vi "Main Window.vi"() -> ()   [LabVIEW 2015]
uses:
  Control Button/Exit.ctl
  Control Button/login.ctl
  Control Button/Logout.ctl
  Control Button/setting.ctl
  Control Button/report.ctl
  Control Button/Manual.ctl
  Control Button/Start.ctl
  Enqueue/Main window Seq/Test selection_1.ctl
  Enqueue/Main window Seq/Test seq_1.ctl
  Galobal variable_TI.vi
  Project Setup/Globle Variable/GR_Servo.vi
panel:
  out "User Name":string
  out "error out":errorcluster
  out "x = y?":bool
  out "Company Name":string
  in  "Sign In":T1
  out "Boolean":bool
  in  "Dashbord":T6
  in  "Login Window":T8 {"User Name" items=["admin", "mmum", "a", "AJAY Kumar", "", "", "", "", "", "", "", "", "", "", "", "", "", "", "", "", "", "", "", "", "", "", "", "", "", "", "", ""]}
  in  "Exit":T9
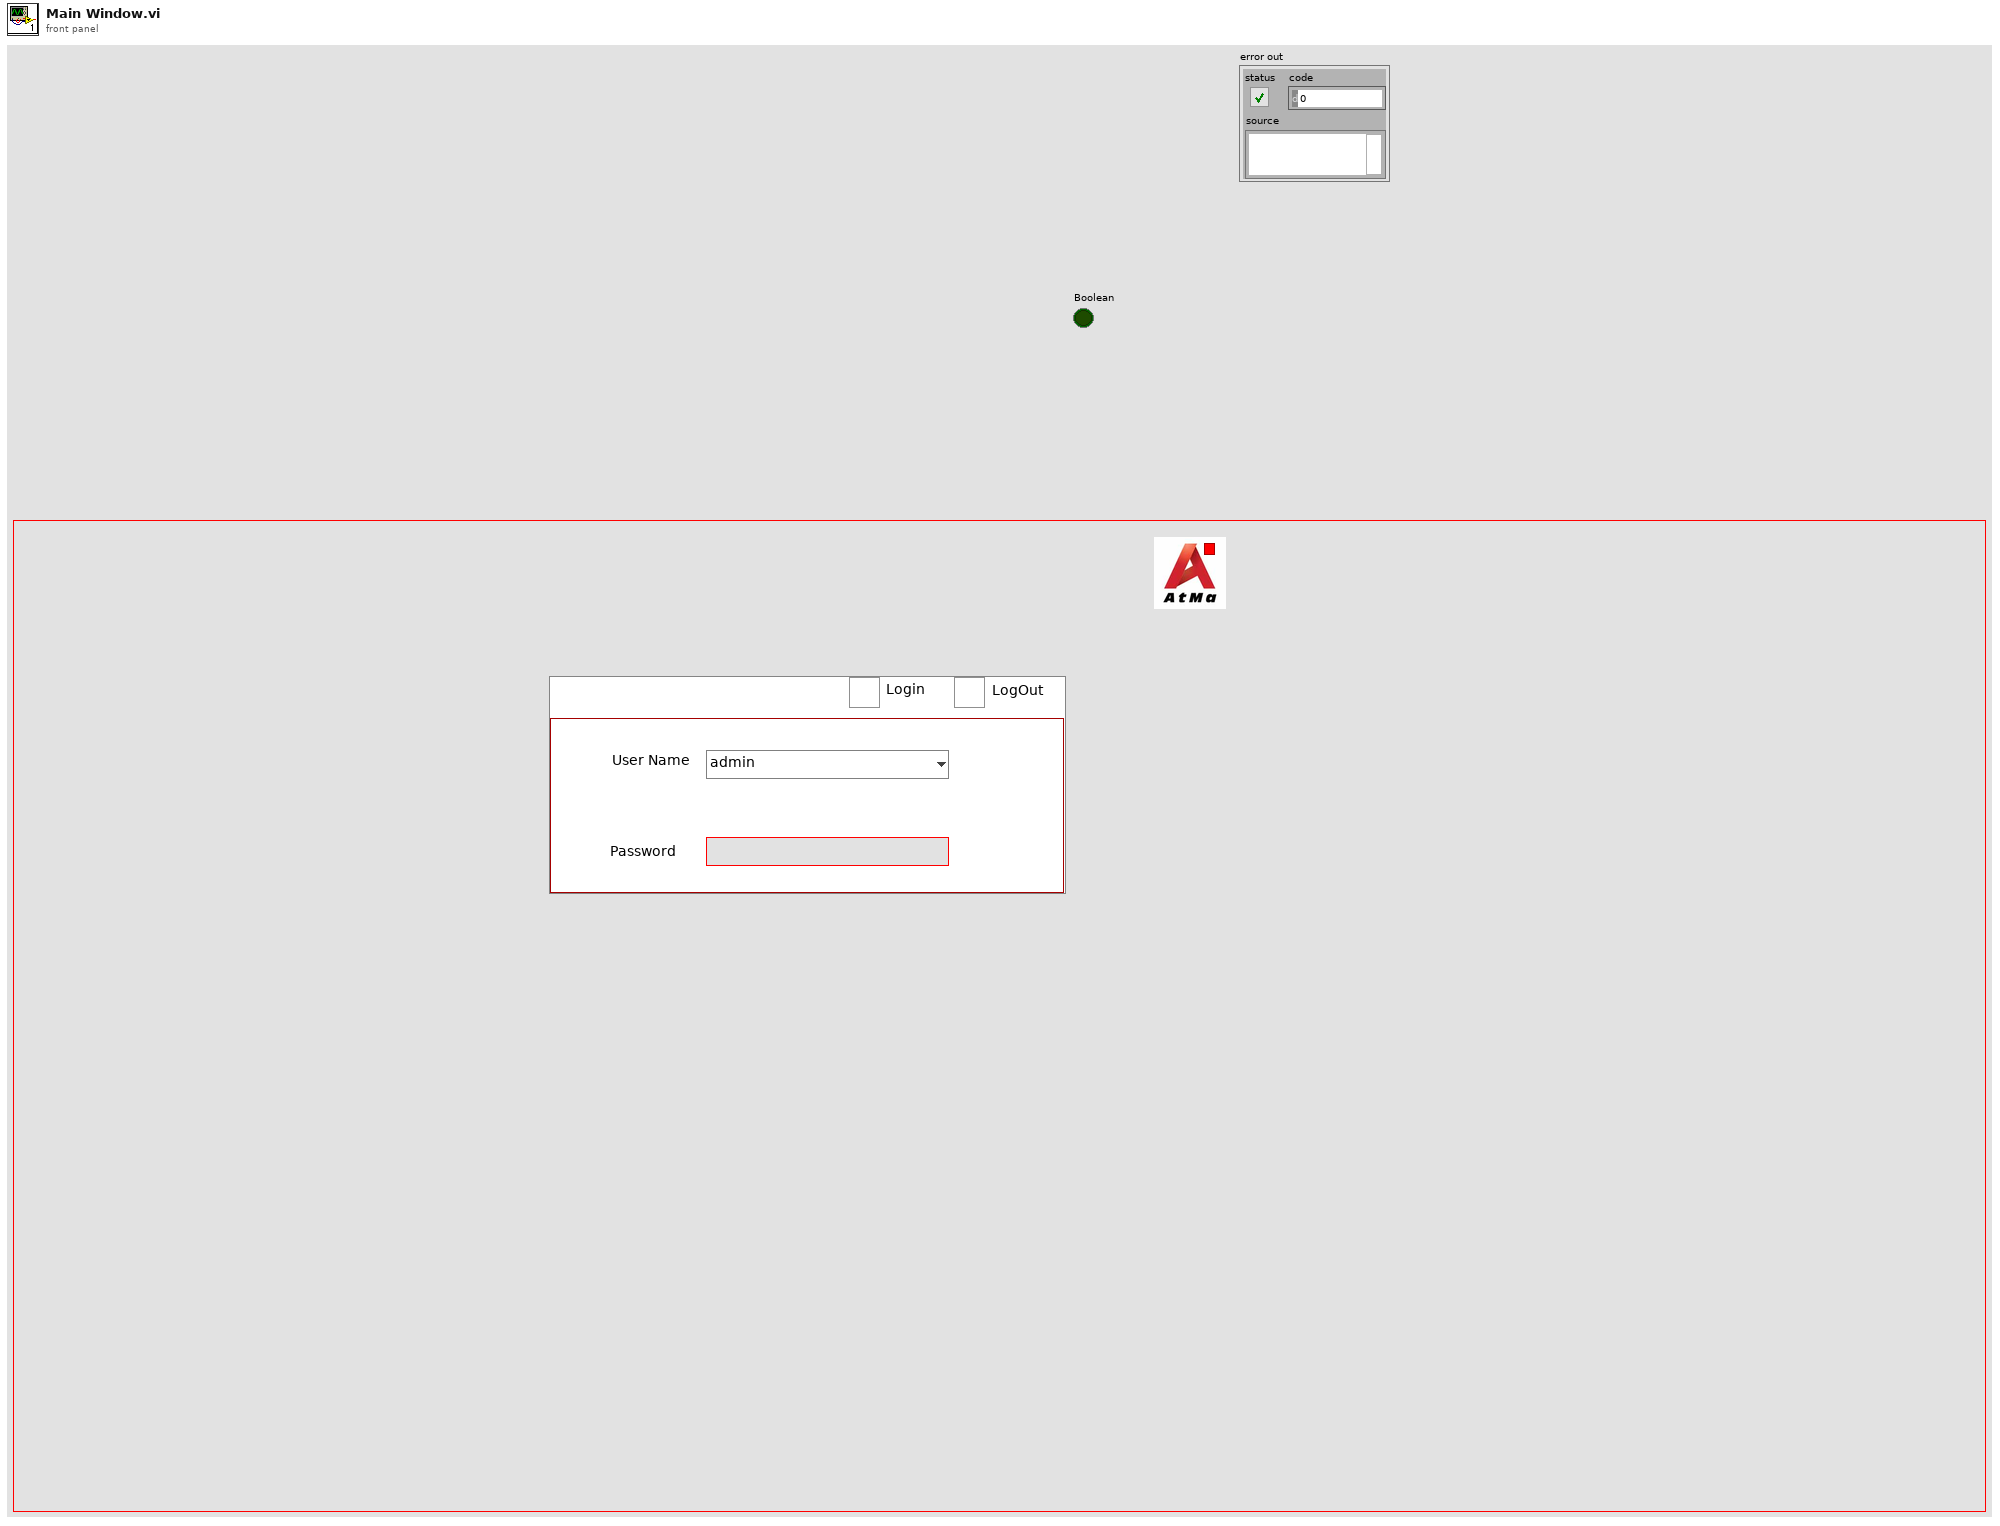
[diagram p1: front panel]
types:
  T1 = typedef "login.ctl" = bool
  T2 = typedef "setting.ctl" = bool
  T3 = typedef "report.ctl" = bool
  T4 = typedef "Manual.ctl" = bool
  T5 = typedef "Start.ctl" = bool
  T6 = cluster{"Setting":T2, "Report":T3, "Manaul":T4, "Start":T5}
  T7 = typedef "Logout.ctl" = bool
  T8 = cluster{"User Name":u16, "Password":string, "Sign In":T1, "Log Out":T7}
  T9 = typedef "Exit.ctl" = bool
  T10 = typedef "Test selection_1.ctl" = enum16{"Init", "Enqueue ", "Enqueue N", "Enqueue in stack", "Enqueue in stack N", "Dequeue", "Dequeue N", "Flush", "Release Queue"}
  T11 = typedef "Test seq_1.ctl" = enum16{"Poll Event", "Login", "Logout", "Confi", "Manual", "Report", "Testing", "Exit"}
  T12 = cluster{"XInput":dbl[], "Y New Value":dbl[], "Avg point":i16}[]
  T13 = cluster{"Slop":dbl[], "Intercept":dbl[], "Average ":i16[]}
  T14 = cluster{"UserName":string[], "Password":string[], "Usertype":string[], "Analog Min":string[], "Analog Max":string[], "DigitalInput Port":string[], "Digital Output Port":string[], "ANalog Port":string[], "IOList":cluster{"DI List_280":string[], "D0List _280":string[], "AI List_280":string[]}}
  T15 = cluster{"DI List_280":string[], "D0List _280":string[], "AI List_280":string[]}
  T16 = cluster{"DigitalInput Port[0]":string, "DigitalInput Port[1]":string, "DigitalInput Port[2]":string, "DigitalInput Port[3]":string, "DigitalInput Port[4]":string, "DigitalInput Port[5]":string, "DigitalInput Port[6]":string, "DigitalInput Port[7]":string, "DigitalInput Port[8]":string, "DigitalInput Port[9]":string, "DigitalInput Port[10]":string, "DigitalInput Port[11]":string, "DigitalInput Port[12]":string, "DigitalInput Port[13]":string, "DigitalInput Port[14]":string, "DigitalInput Port[15]":string}
  T17 = cluster{"Digital Output Port[0]":string, "Digital Output Port[1]":string, "Digital Output Port[2]":string, "Digital Output Port[3]":string, "Digital Output Port[4]":string, "Digital Output Port[5]":string, "Digital Output Port[6]":string, "Digital Output Port[7]":string, "Digital Output Port[8]":string, "Digital Output Port[9]":string, "Digital Output Port[10]":string, "Digital Output Port[11]":string, "Digital Output Port[12]":string, "Digital Output Port[13]":string, "Digital Output Port[14]":string, "Digital Output Port[15]":string, "Digital Output Port[16]":string, "Digital Output Port[17]":string, "Digital Output Port[18]":string, "Digital Output Port[19]":string, "Digital Output Port[20]":string, "Digital Output Port[21]":string, "Digital Output Port[22]":string, "Digital Output Port[23]":string, "Digital Output Port[24]":string, "Digital Output Port[25]":string, "Digital Output Port[26]":string, "Digital Output Port[27]":string, "Digital Output Port[28]":string, "Digital Output Port[29]":string}
  T18 = cluster{"ANalog Port[0]":string, "ANalog Port[1]":string, "ANalog Port[2]":string, "ANalog Port[3]":string, "ANalog Port[4]":string, "ANalog Port[5]":string, "ANalog Port[6]":string, "ANalog Port[7]":string, "ANalog Port[8]":string, "ANalog Port[9]":string, "ANalog Port[10]":string, "ANalog Port[11]":string, "ANalog Port[12]":string, "ANalog Port[13]":string, "ANalog Port[14]":string, "ANalog Port[15]":string, "ANalog Port[16]":string, "ANalog Port[17]":string, "ANalog Port[18]":string, "ANalog Port[19]":string, "ANalog Port[20]":string, "ANalog Port[21]":string, "ANalog Port[22]":string, "ANalog Port[23]":string, "ANalog Port[24]":string, "ANalog Port[25]":string, "ANalog Port[26]":string, "ANalog Port[27]":string, "ANalog Port[28]":string, "ANalog Port[29]":string, "ANalog Port[30]":string, "ANalog Port[31]":string}
  T19 = enum32{"Invalid", "Standard", "Closed", "Hidden", "Minimized", "Maximized"}
  T20 = enum8{"Enabled", "Disabled", "Disabled and Grayed Out"}
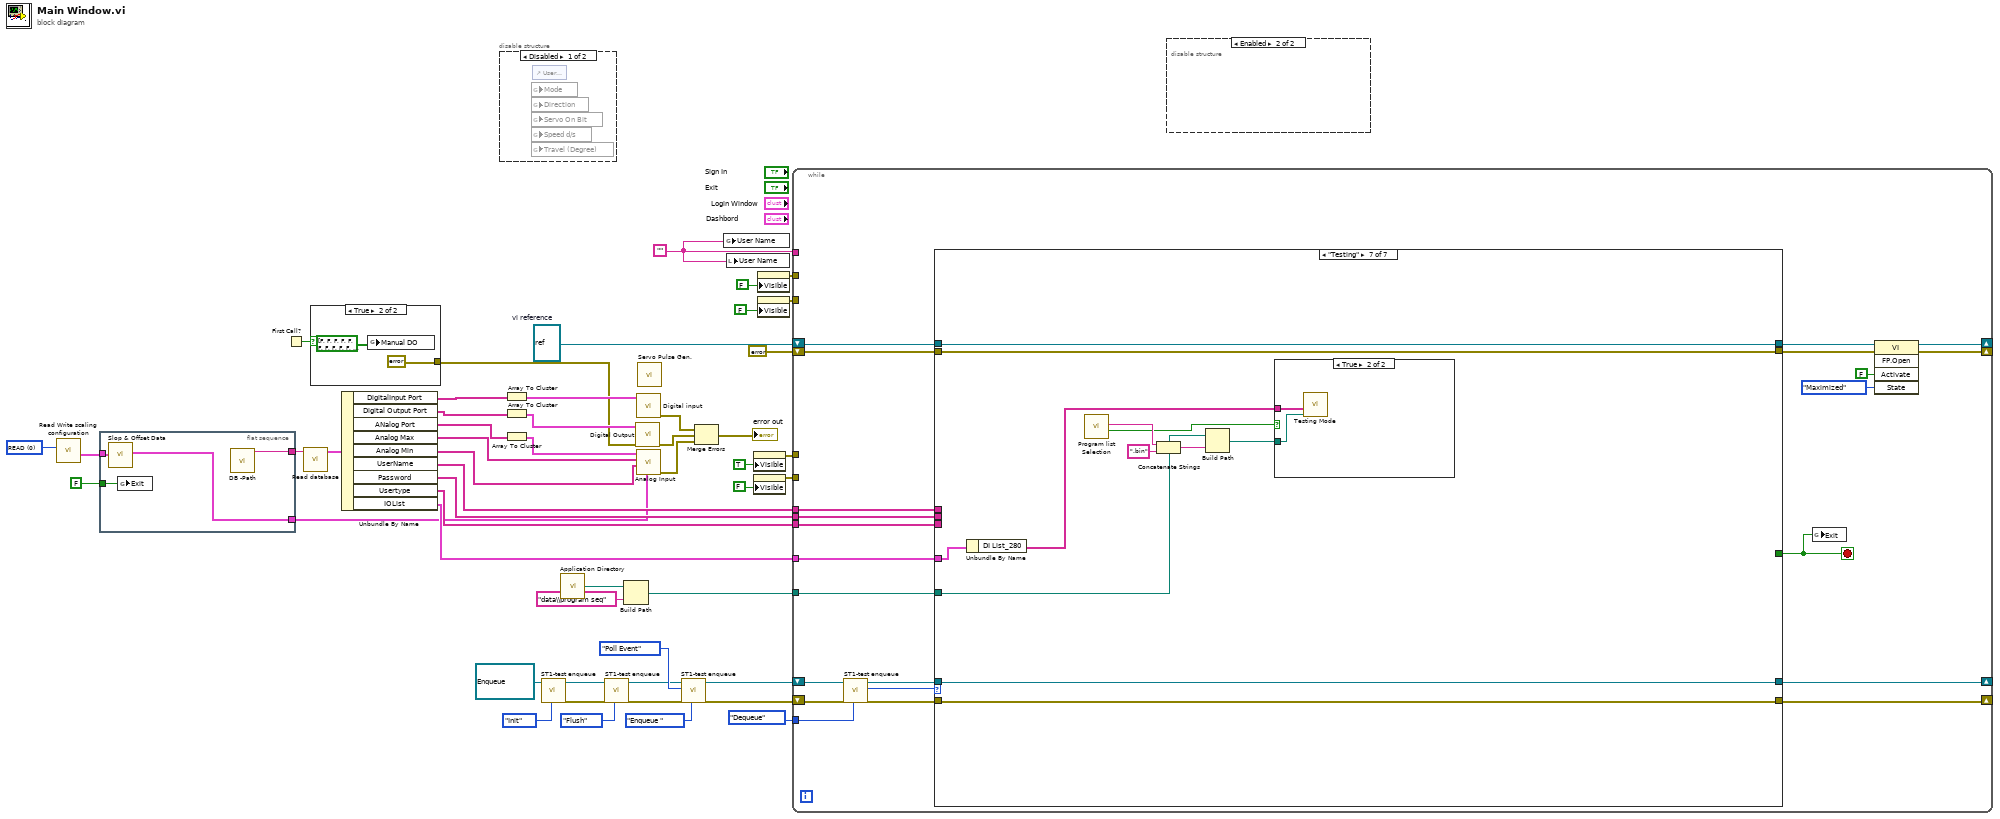
[diagram p0: block diagram]
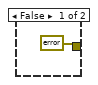
[diagram p2: hidden frame]
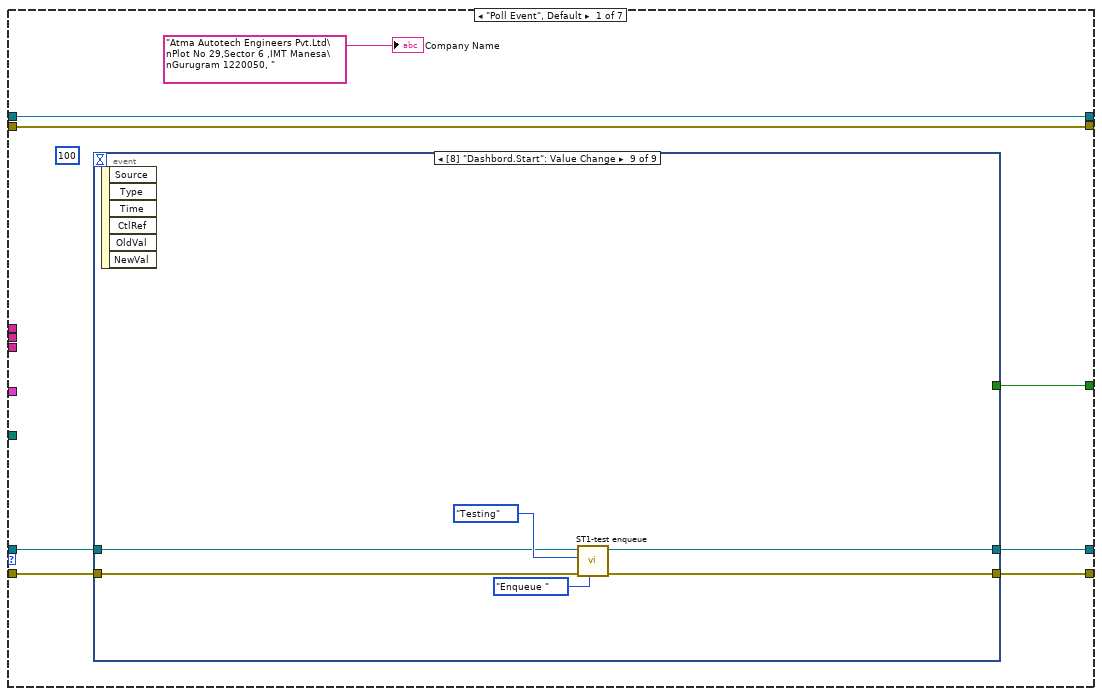
[diagram p5: hidden frame]
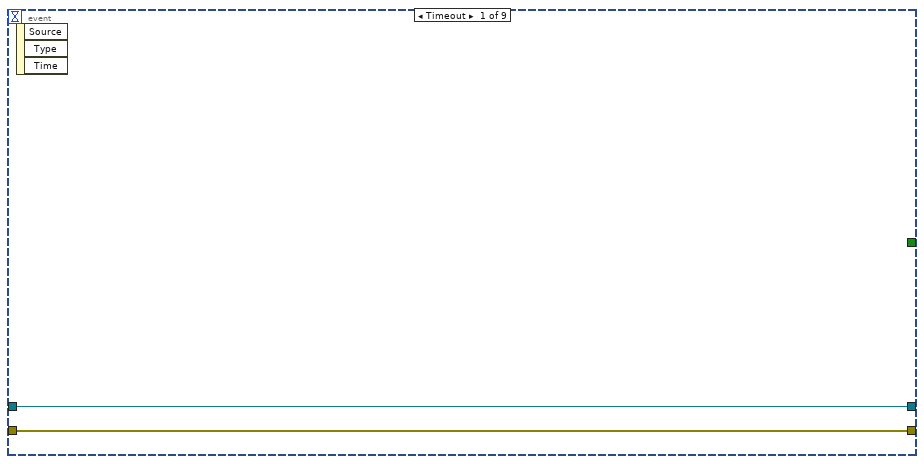
[diagram p6: hidden frame]
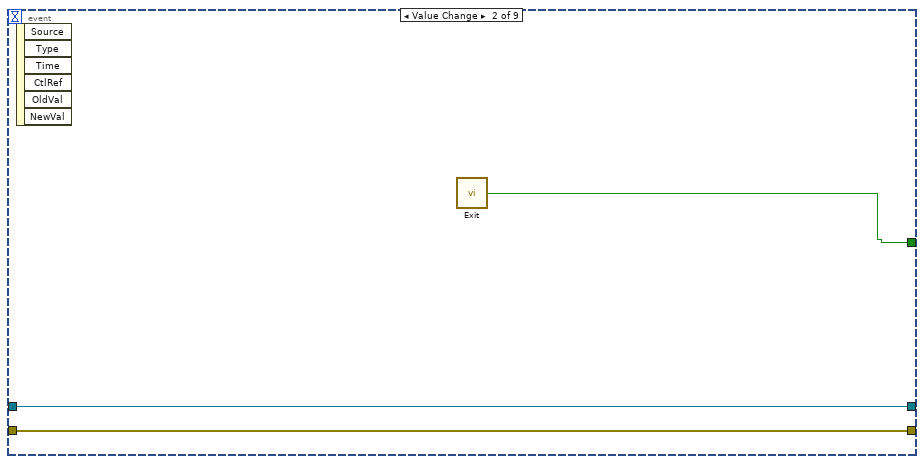
[diagram p7: hidden frame]
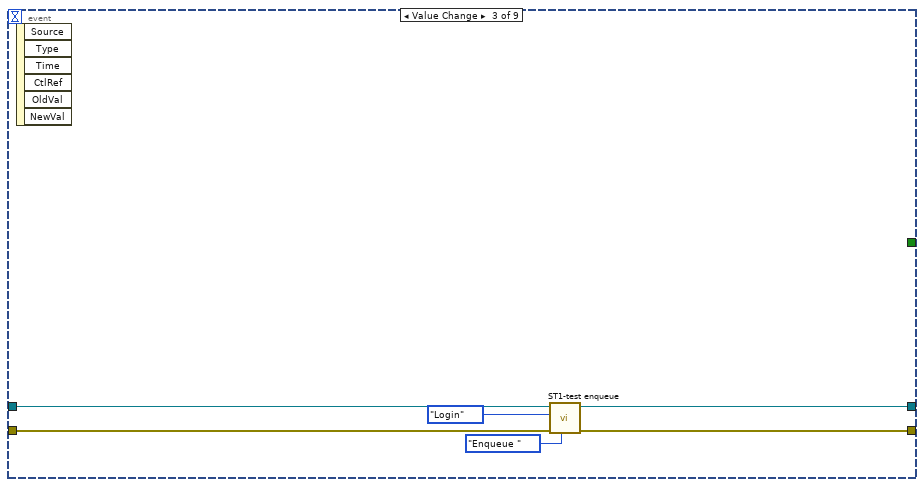
[diagram p8: hidden frame]
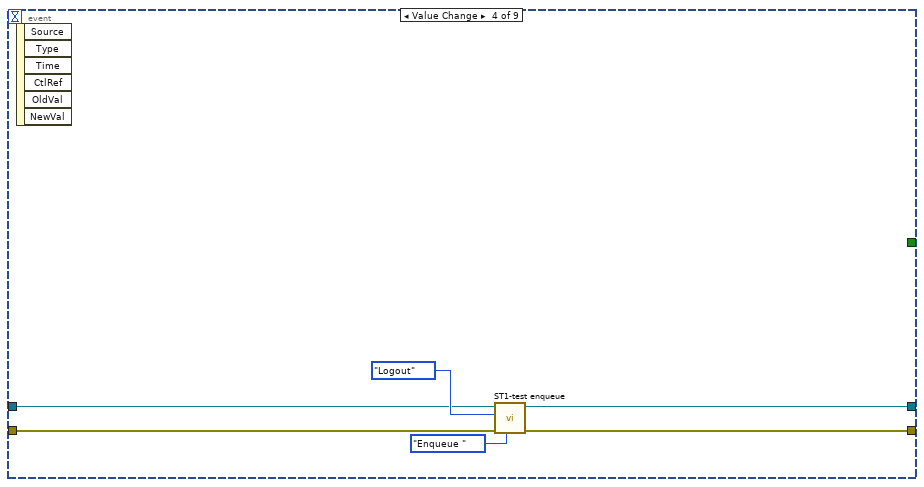
[diagram p9: hidden frame]
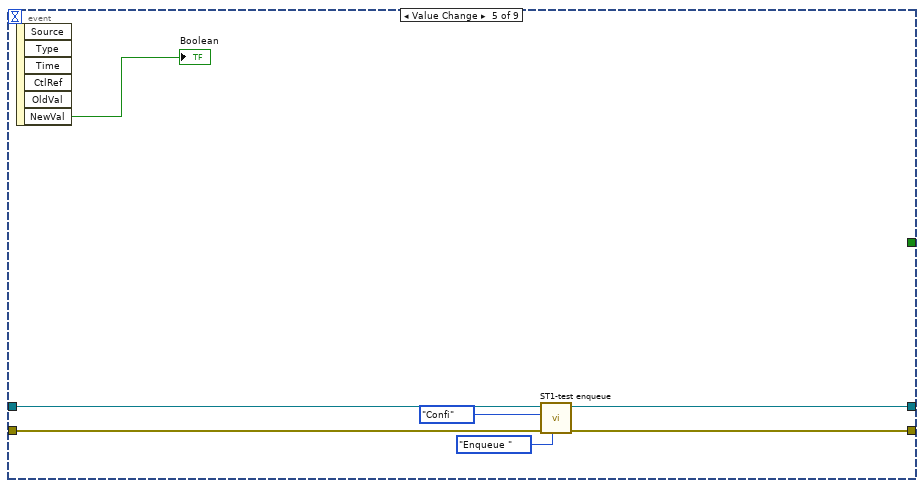
[diagram p10: hidden frame]
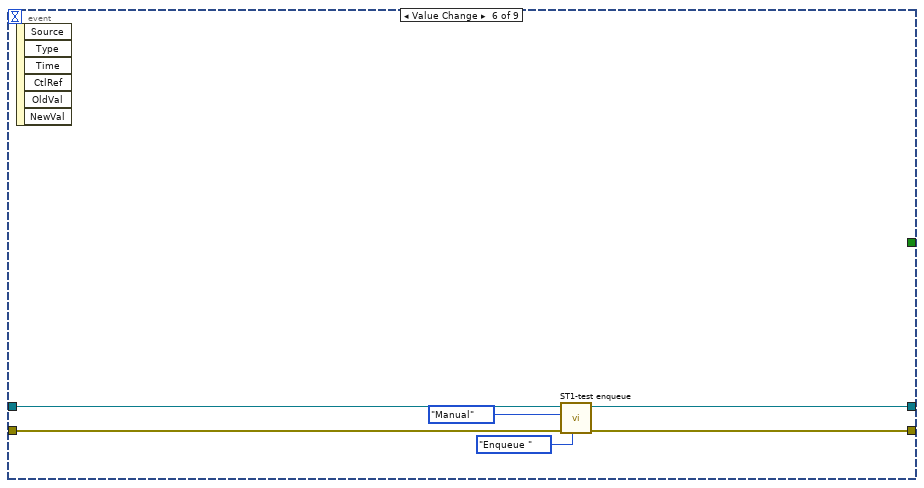
[diagram p11: hidden frame]
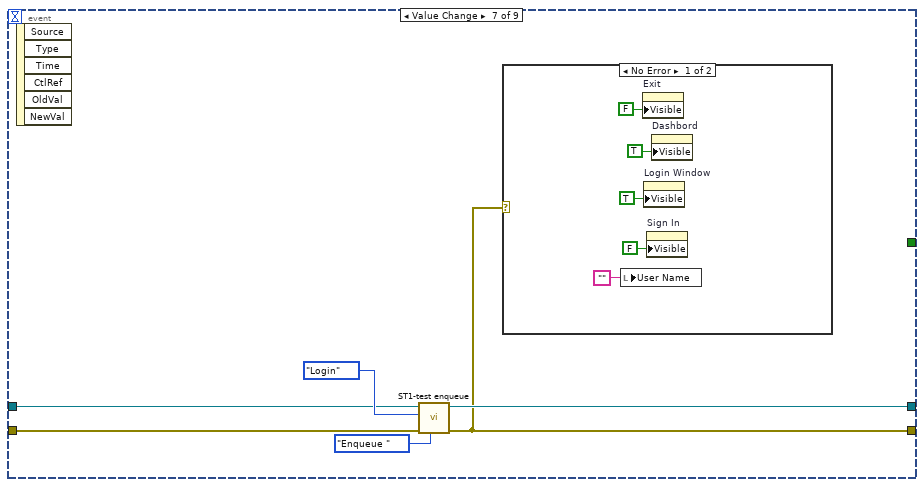
[diagram p12: hidden frame]
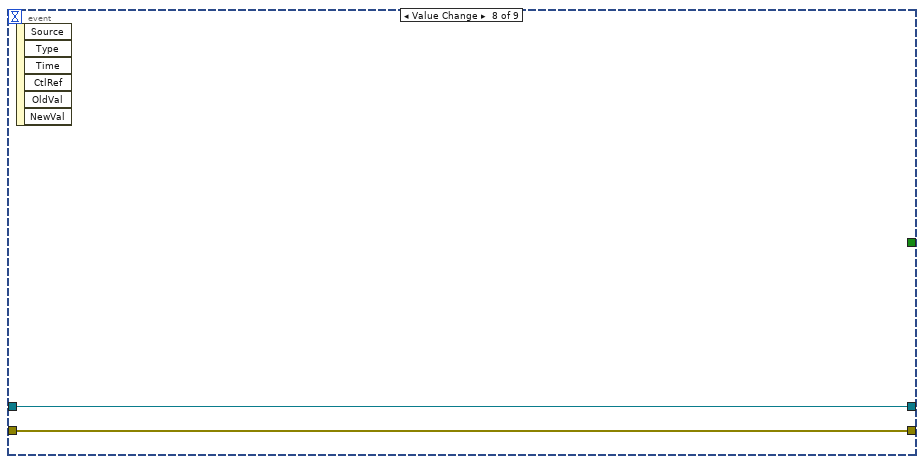
[diagram p14: hidden frame]
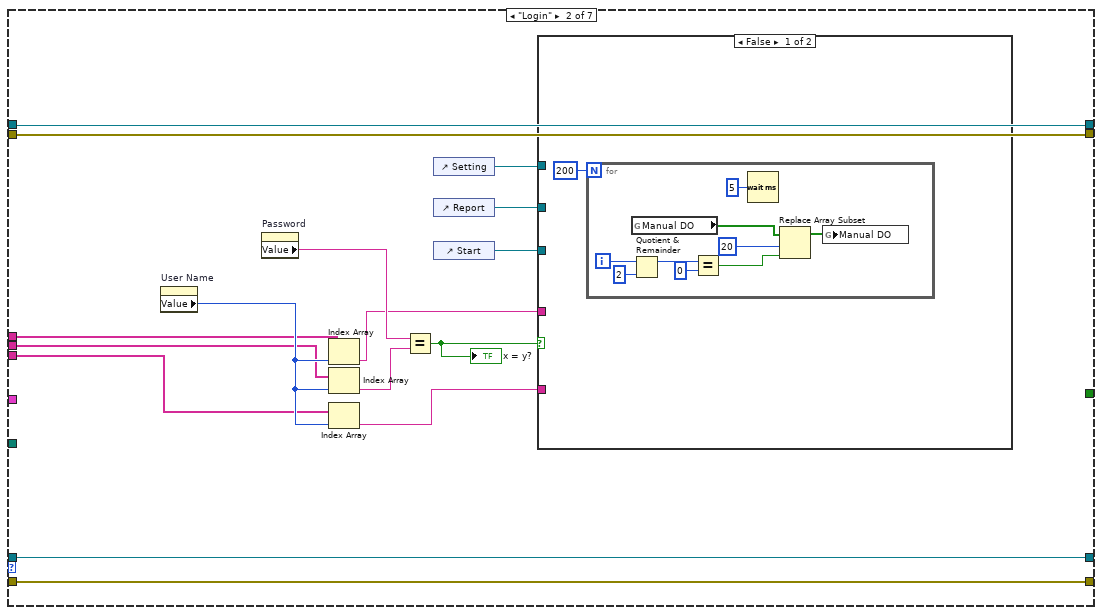
[diagram p15: hidden frame]
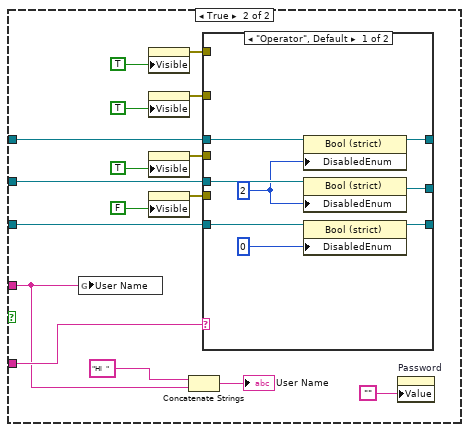
[diagram p16: hidden frame]
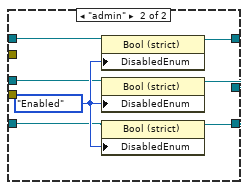
[diagram p17: hidden frame]
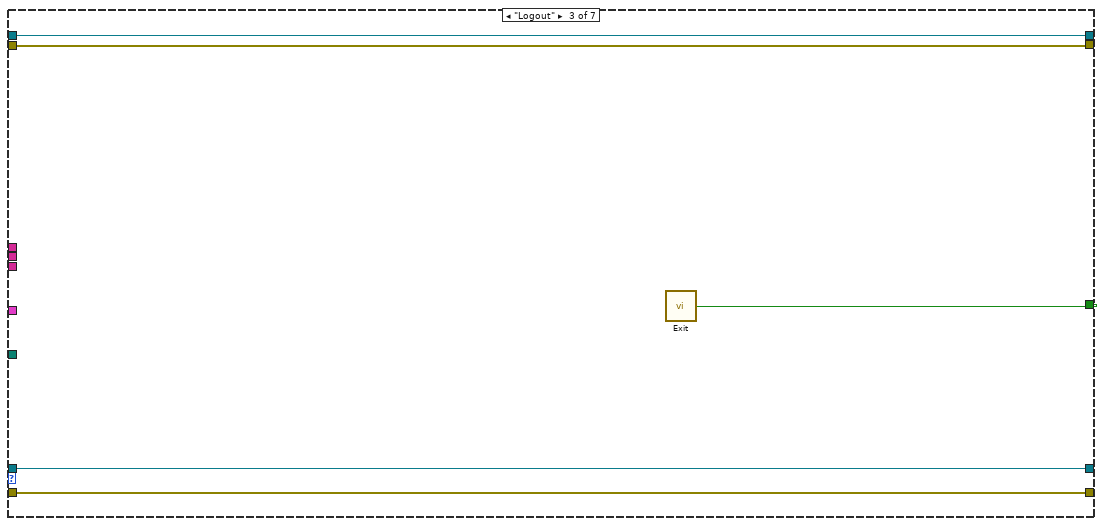
[diagram p18: hidden frame]
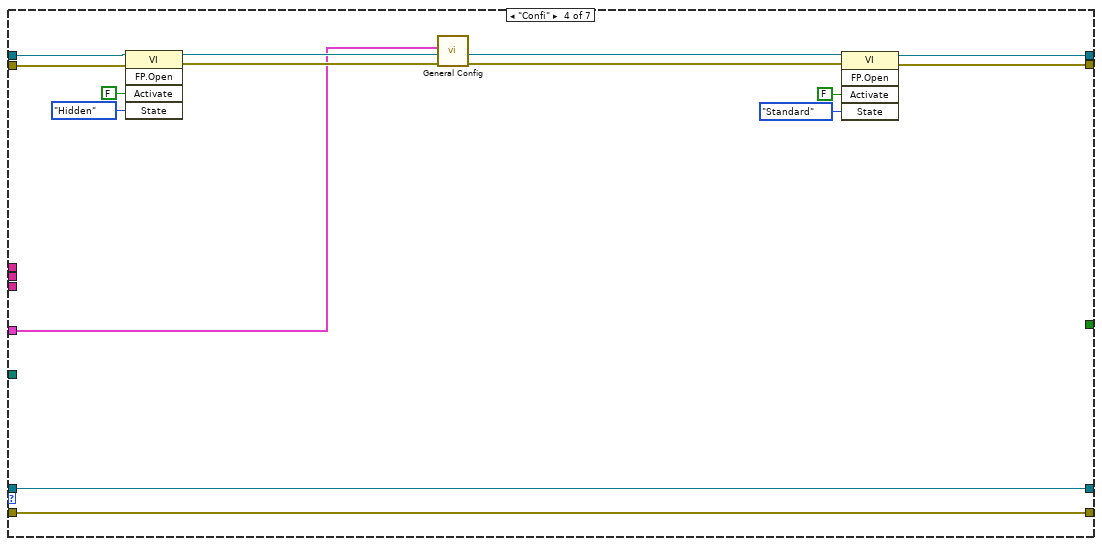
[diagram p19: hidden frame]
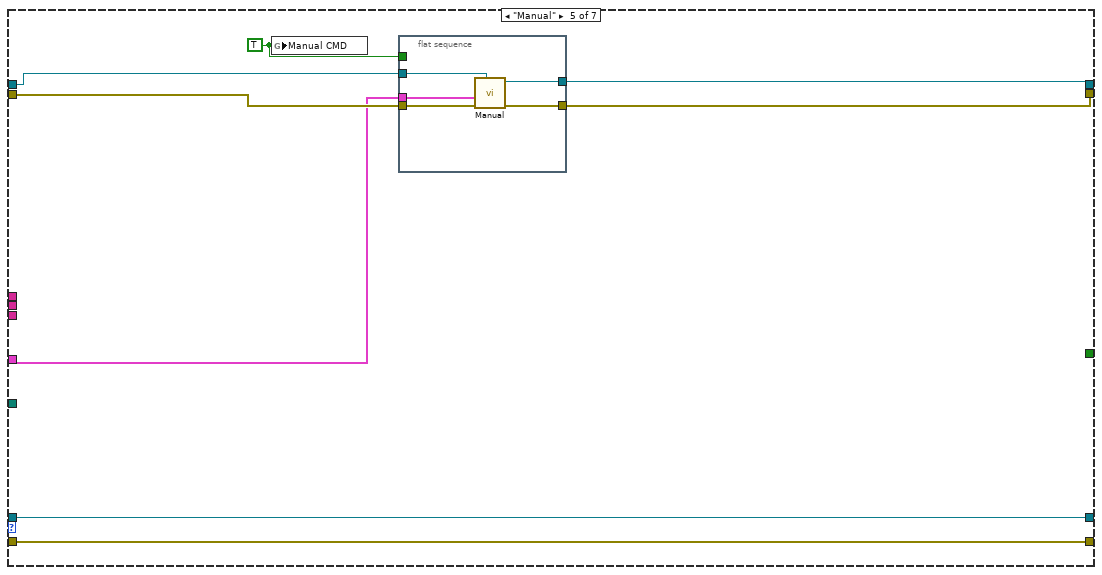
[diagram p20: hidden frame]
diagram:
  w13 = u16 0 items=["READ", "WRITE"] ("Read/Write")
  w28 = ""
  w38 = refnum<vi> refnum  # vi reference
  w39 = refnum<queue> refnum items=["Poll Event", "Login", "Logout", "Confi", "Manual", "Report", "Testing", "Exit"] ("queue in")
  n1 = call "Read Write scaling configuration.vi"("Read/Write"=w13) -> ("Output"=w12:T12)  [unwired: 4 in, 2 out]
  n2 = flat-sequence {
    tunnel: [w54] -> w27
    tunnel: w12 -> [w53]
    tunnel: [w52] -> w11
    tunnel: FALSE ("Exit") -> [w51]
    frame #0 {
      n3 = call "Slop & Offset Data.vi"("Input"=w53) -> ("Cluster"=w52:T13)  [unwired: 10 in]
      n4 = global write "Galobal variable_TI.vi" "Exit"(w51) -> ()
      n5 = call "DB -Path.vi"() -> ("String"=w54:string)  [unwired: 11 in]
    }
  }
  n6 = First Call?() -> (First Call?: T/F=w2:bool)
  n7 = call "Read database.vi"("String"=w27) -> ("DB Data"=w26:T14)  [unwired: 3 in, 1 out]
  n8 = case shown="True" w2 {
    tunnel: [errorcluster {"status"=FALSE, "code"=0, "source"=""} ("error constant") errorcluster {"status"=FALSE, "code"=0, "source"=""} ("error constant")] -> w1
    frame False {
    }
    frame True {
      n9 = global write "Galobal variable_TI.vi" "Manual DO"(bool[] [FALSE, FALSE, FALSE, FALSE, FALSE, FALSE, FALSE, FALSE, FALSE, FALSE, FALSE, FALSE, FALSE, FALSE, FALSE, FALSE, FALSE, FALSE, FALSE, FALSE, FALSE, FALSE, FALSE, FALSE, FALSE, FALSE, FALSE, FALSE, FALSE, FALSE] ("Manual DO")) -> ()
    }
  }
  n10 = Unbundle By Name(w26) -> ("DigitalInput Port"=w25:string[], "Digital Output Port"=w23:string[], "ANalog Port"=w21:string[], "Analog Max"=w19:string[], "Analog Min"=w18:string[], "UserName"=w17:string[], "Password"=w16:string[], "Usertype"=w15:string[], "IOList"=w14:T15)
  n11 = disable-structure shown="Disabled" {
    frame Disabled {
      n12 = global read "GR_Servo.vi" "Mode"() -> ()  [unwired: 1 in]
      n13 = global read "GR_Servo.vi" "Direction"() -> ()  [unwired: 1 in]
      n14 = global read "GR_Servo.vi" "Servo On Bit"() -> ()  [unwired: 1 in]
      n15 = global read "GR_Servo.vi" "Speed d/s"() -> ()  [unwired: 1 in]
      n16 = global read "GR_Servo.vi" "Travel (Degree)"() -> ()  [unwired: 1 in]
      n17 = control-ref of="User Name"() -> ()  [unwired: 1 out]
    }
    frame Enabled {
    }
  }
  n18 = Array To Cluster(array=w25) -> (cluster=w24:T16)
  n19 = Array To Cluster(array=w23) -> (cluster=w22:T17)
  n20 = Array To Cluster(array=w21) -> (cluster=w20:T18)
  n21 = call "ST1-test enqueue.vi"("Enum Selection"=Test_selection_1."Init", "queue in"=w39) -> ("error out"=w48:errorcluster, "queue Out"=w44:refnum<queue>)  [unwired: 6 in, 1 out]
  n22 = call <vilib>:"Application Directory.vi"() -> ("Application Directory"=w5:path)
  n23 = call "ST1-test enqueue.vi"("Enum Selection"=Test_selection_1."Flush", "Error In"=w48, "queue in"=w44) -> ("error out"=w46:errorcluster, "queue Out"=w43:refnum<queue>)  [unwired: 5 in, 1 out]
  n24 = Build Path(base path=w5, name or relative path="data\\program seq") -> (appended path=w3:path)
  n25 = call "Digital Output.vi"("error in"=w1, "DAQmx OutPut Setting"=w22) -> ("error out"=w9:errorcluster)  [unwired: 8 in, 1 out]
  n26 = call "Digital input.vi"("DAQmx InPut Setting"=w24) -> ("error out"=w7:errorcluster)  [unwired: 9 in, 1 out]
  n27 = call "Analog Input.vi"("clai. Parmeter"=w11, "Min Value"=w18, "Max Value"=w19, "DAQmx Analog Input Setting"=w20) -> ("error out"=w8:errorcluster)  [unwired: 6 in, 1 out]
  n28 = call "Servo Pulse Gen..vi"() -> ()  [unwired: 12 in]
  n29 = call "ST1-test enqueue.vi"("Enum Selection"=Test_selection_1."Enqueue ", "Error In"=w46, "Enqueue"=Test_seq_1."Poll Event", "queue in"=w43) -> ("error out"=w41:errorcluster, "queue Out"=w42:refnum<queue>)  [unwired: 4 in, 1 out]
  n30 = Merge Errors(w7, w9, w8) -> (→"error out":errorcluster)
  n31 = global write "Galobal variable_TI.vi" "User Name"(w28) -> ()
  n32 = local write "User Name"(w28) -> ()
  n33 = property on="Login Window" class="Clust (strict)"("Visible"=TRUE) -> (error out=w33:errorcluster)  [unwired: 2 in, 1 out]
  n34 = property on="Sign In" class="Bool (strict)"("Visible"=FALSE) -> (error out=w32:errorcluster)  [unwired: 2 in, 1 out]
  n35 = property on="Exit" class="Bool (strict)"("Visible"=FALSE) -> (error out=w30:errorcluster)  [unwired: 2 in, 1 out]
  n36 = property on="Dashbord" class="Clust (strict)"("Visible"=FALSE) -> (error out=w35:errorcluster)  [unwired: 2 in, 1 out]
  n37 = while {
    shift-right: [w73] -> _
    shift-left: w42 -> [w79]
    shift-right: [w72] -> _
    shift-left: w41 -> [w78]
    tunnel: Test_selection_1."Dequeue" ("Enum Selection") -> [w77]
    shift-right: [w64] -> _
    shift-left: errorcluster {"status"=FALSE, "code"=0, "source"=""} ("error out") -> [w70]
    shift-right: [w65] -> _
    shift-left: w38 -> [w71]
    tunnel: w35 -> [_]
    tunnel: w33 -> [_]
    tunnel: w32 -> [_]
    tunnel: w30 -> [_]
    tunnel: w28 -> [_]
    tunnel: w17 -> [w63]
    tunnel: w16 -> [w62]
    tunnel: w15 -> [w61]
    tunnel: w14 -> [w60]
    tunnel: w3 -> [w58]
    stop <- w59 stop-if-true
    n38 = call "ST1-test enqueue.vi"("Enum Selection"=w77, "Error In"=w78, "queue in"=w79) -> ("error out"=w74:errorcluster, "D-enqueue"=w76:T11, "queue Out"=w75:refnum<queue>)  [unwired: 5 in]
    n39 = case shown="\"Testing\"" w76 {
      tunnel: [w85 _ w194 _ _ _ _] -> w59
      tunnel: w75 -> [w86 w152 w198 w212 w220 w229 w241]
      tunnel: w74 -> [w87 w151 w197 w211 w219 w228 w240]
      tunnel: [w84 w152 w198 w212 w220 w229 w241] -> w73
      tunnel: [w83 w151 w197 w211 w219 w228 w240] -> w72
      tunnel: [w82 w143 w196 w206 w215 w227 w239] -> w67
      tunnel: [w81 w142 w195 w205 w216 w226 w238] -> w66
      tunnel: w71 -> [w82 w143 w196 w204 w217 w227 w239]
      tunnel: w70 -> [w81 w142 w195 w203 w218 w226 w238]
      tunnel: w63 -> [_ w140 _ _ _ _ _]
      tunnel: w62 -> [_ w139 _ _ _ _ _]
      tunnel: w61 -> [_ w138 _ _ _ _ _]
      tunnel: w60 -> [_ _ _ w199 w214 _ w232]
      tunnel: w58 -> [_ _ _ _ _ _ w234]
      frame "Poll Event", Default {
        (unwired) 100
        n40 = event shown="[8] \"Dashbord.Start\": Value Change" {
          selector: _ -> [_ _ _ _ _ _ _ _ _]
          dyn-events: _ -> [_ _ _ _ _ _ _ _ _]
          timeout: _ -> [_ _ _ _ _ _ _ _ _]
          tunnel: [_ w90 _ _ _ _ _ _ _] -> w85
          tunnel: w87 -> [w88 w91 w96 w99 w107 w115 w121 w129 w133]
          tunnel: w86 -> [w89 w92 w97 w100 w108 w113 w120 w130 w134]
          tunnel: [w89 w92 w95 w102 w106 w112 w119 w130 w132] -> w84
          tunnel: [w88 w91 w94 w101 w105 w114 w118 w129 w131] -> w83
          event Timeout {
            n41 = event-data() -> ()  [unwired: 1 in, 3 out]
          }
          event Value Change {
            n42 = event-data() -> ()  [unwired: 1 in, 6 out]
            n43 = call "Exit.vi"() -> ("Exit"=w90:bool)  [unwired: 1 in]
          }
          event Value Change {
            n44 = event-data() -> ()  [unwired: 1 in, 6 out]
            n45 = call "ST1-test enqueue.vi"("Enum Selection"=Test_selection_1."Enqueue ", "Error In"=w96, "Enqueue"=Test_seq_1."Login", "queue in"=w97) -> ("error out"=w94:errorcluster, "queue Out"=w95:refnum<queue>)  [unwired: 4 in, 1 out]
          }
          event Value Change {
            n46 = event-data() -> ()  [unwired: 1 in, 6 out]
            n47 = call "ST1-test enqueue.vi"("Enum Selection"=Test_selection_1."Enqueue ", "Error In"=w99, "Enqueue"=Test_seq_1."Logout", "queue in"=w100) -> ("error out"=w101:errorcluster, "queue Out"=w102:refnum<queue>)  [unwired: 4 in, 1 out]
          }
          event Value Change {
            n48 = event-data() -> ("NewVal"=→"Boolean":T2)  [unwired: 1 in, 5 out]
            n49 = call "ST1-test enqueue.vi"("Enum Selection"=Test_selection_1."Enqueue ", "Error In"=w107, "Enqueue"=Test_seq_1."Confi", "queue in"=w108) -> ("error out"=w105:errorcluster, "queue Out"=w106:refnum<queue>)  [unwired: 4 in, 1 out]
          }
          event Value Change {
            n50 = event-data() -> ()  [unwired: 1 in, 6 out]
            n51 = call "ST1-test enqueue.vi"("Enum Selection"=Test_selection_1."Enqueue ", "Error In"=w115, "Enqueue"=Test_seq_1."Manual", "queue in"=w113) -> ("error out"=w114:errorcluster, "queue Out"=w112:refnum<queue>)  [unwired: 4 in, 1 out]
          }
          event Value Change {
            n52 = event-data() -> ()  [unwired: 1 in, 6 out]
            n53 = call "ST1-test enqueue.vi"("Enum Selection"=Test_selection_1."Enqueue ", "Error In"=w121, "Enqueue"=Test_seq_1."Login", "queue in"=w120) -> ("error out"=w118:errorcluster, "queue Out"=w119:refnum<queue>)  [unwired: 4 in, 1 out]
            n54 = case shown="No Error" w118 {
              frame No Error {
                n55 = local write "User Name"("") -> ()
                n56 = property on="Exit" class="Bool (strict)"("Visible"=FALSE) -> ()  [unwired: 2 in, 2 out]
                n57 = property on="Login Window" class="Clust (strict)"("Visible"=TRUE) -> ()  [unwired: 2 in, 2 out]
                n58 = property on="Sign In" class="Bool (strict)"("Visible"=FALSE) -> ()  [unwired: 2 in, 2 out]
                n59 = property on="Dashbord" class="Clust (strict)"("Visible"=TRUE) -> ()  [unwired: 2 in, 2 out]
              }
              frame Error {
              }
            }
          }
          event Value Change {
            n60 = event-data() -> ()  [unwired: 1 in, 6 out]
          }
          event Value Change {
            n61 = event-data() -> ()  [unwired: 1 in, 6 out]
            n62 = call "ST1-test enqueue.vi"("Enum Selection"=Test_selection_1."Enqueue ", "Error In"=w133, "Enqueue"=Test_seq_1."Testing", "queue in"=w134) -> ("error out"=w131:errorcluster, "queue Out"=w132:refnum<queue>)  [unwired: 4 in, 1 out]
          }
        }
        "Company Name" <- "Atma Autotech Engineers Pvt.Ltd\nPlot No 29,Sector 6 ,IMT Manesa\nGurugram 1220050, " ("string")
      }
      frame "Login" {
        n63 = property on="User Name" class="Ring (strict)"() -> ("Value"=w150:u16)  [unwired: 2 in, 2 out]
        n64 = property on="Password" class="Str"() -> ("Value"=w148:string)  [unwired: 2 in, 2 out]
        n65 = Index Array(array=w140, index=w150) -> (element=w141:string)
        n66 = Index Array(array=w139, index=w150) -> (element=w149:string)
        n67 = Index Array(array=w138, index=w150) -> (element=w147:string)
        n68 = Equal?(x=w148, y=w149) -> (x = y?=w137:bool)
        "x = y?" <- w137
        n69 = control-ref of="Setting"() -> (w146:refnum<vi>)
        n70 = control-ref of="Report"() -> (w144:refnum<vi>)
        n71 = control-ref of="Start"() -> (w145:refnum<vi>)
        n72 = case shown="False" w137 {
          tunnel: w147 -> [_ w174]
          tunnel: w146 -> [_ w178]
          tunnel: w144 -> [_ w177]
          tunnel: w145 -> [_ w176]
          tunnel: w141 -> [_ w163]
          frame False {
            n73 = for {
              N: 200 -> [_]
              i -> [w162]
              n74 = global read "Galobal variable_TI.vi" "Manual DO"() -> (w157:bool[])
              n75 = Quotient & Remainder(x=w162, y=2) -> (x-y*floor(x/y)=w160:i32)  [unwired: 1 out]
              n76 = Equal?(x=w160, y=0) -> (x = y?=w156:bool)
              n77 = Wait (ms)(milliseconds to wait=u32 5) -> ()  [unwired: 1 out]
              n78 = Replace Array Subset(array=w157, new element=w156, index=20) -> (w154:bool[])
              n79 = global write "Galobal variable_TI.vi" "Manual DO"(w154) -> ()
            }
          }
          frame True {
            n80 = global write "Galobal variable_TI.vi" "User Name"(w163) -> ()
            n81 = property on="Exit" class="Bool (strict)"("Visible"=TRUE) -> (error out=w165:errorcluster)  [unwired: 2 in, 1 out]
            n82 = property on="Dashbord" class="Clust (strict)"("Visible"=TRUE) -> (error out=w170:errorcluster)  [unwired: 2 in, 1 out]
            n83 = property on="Sign In" class="Bool (strict)"("Visible"=TRUE) -> (error out=w169:errorcluster)  [unwired: 2 in, 1 out]
            n84 = property on="Login Window" class="Clust (strict)"("Visible"=FALSE) -> (error out=w171:errorcluster)  [unwired: 2 in, 1 out]
            n85 = Concatenate Strings("Hi  " ("string"), w163) -> (→"User Name":string)
            n86 = case shown="\"Operator\", Default" w174 {
              tunnel: [w186 w192] -> _
              tunnel: [w185 w191] -> _
              tunnel: [w184 w190] -> _
              tunnel: w178 -> [w183 w189]
              tunnel: w177 -> [w182 w188]
              tunnel: w176 -> [w181 w187]
              tunnel: w171 -> [_ _]
              tunnel: w170 -> [_ _]
              tunnel: w169 -> [_ _]
              tunnel: w165 -> [_ _]
              frame "Operator", Default {
                w179 = 2
                n87 = property class="Bool (strict)"(reference=w183, "DisabledEnum"=w179) -> (reference out=w186:refnum<vi>)  [unwired: 1 in, 1 out]
                n88 = property class="Bool (strict)"(reference=w182, "DisabledEnum"=w179) -> (reference out=w185:refnum<vi>)  [unwired: 1 in, 1 out]
                n89 = property class="Bool (strict)"(reference=w181, "DisabledEnum"=0) -> (reference out=w184:refnum<vi>)  [unwired: 1 in, 1 out]
              }
              frame "admin" {
                w193 = T20."Enabled" ("Disabled")
                n90 = property class="Bool (strict)"(reference=w189, "DisabledEnum"=w193) -> (reference out=w192:refnum<vi>)  [unwired: 1 in, 1 out]
                n91 = property class="Bool (strict)"(reference=w188, "DisabledEnum"=w193) -> (reference out=w191:refnum<vi>)  [unwired: 1 in, 1 out]
                n92 = property class="Bool (strict)"(reference=w187, "DisabledEnum"=w193) -> (reference out=w190:refnum<vi>)  [unwired: 1 in, 1 out]
              }
            }
            n93 = property on="Password" class="Str"("Value"="") -> ()  [unwired: 2 in, 2 out]
          }
        }
      }
      frame "Logout" {
        n94 = call "Exit.vi"() -> ("Exit"=w194:bool)  [unwired: 1 in]
      }
      frame "Confi" {
        n95 = invoke class="VI" method="FP.Open"(reference=w204, error in=w203, "Activate"=FALSE ("Activate?"), "State"=T19."Hidden") -> (reference out=w200:refnum<vi>, error out=w202:errorcluster)  [unwired: 1 in, 3 out]
        n96 = call "General Config.vi"("error In"=w202, "IOList"=w199) -> ("error out"=w201:errorcluster)  [unwired: 8 in, 1 out]
        n97 = invoke class="VI" method="FP.Open"(reference=w200, error in=w201, "Activate"=FALSE ("Activate?"), "State"=T19."Standard") -> (reference out=w206:refnum<vi>, error out=w205:errorcluster)  [unwired: 1 in, 3 out]
      }
      frame "Manual" {
        w213 = TRUE ("Manual CMD")
        n98 = global write "Galobal variable_TI.vi" "Manual CMD"(w213) -> ()
        n99 = flat-sequence {
          tunnel: w218 -> [w225]
          tunnel: w217 -> [w224]
          tunnel: [w223] -> w216
          tunnel: [w222] -> w215
          tunnel: w214 -> [w221]
          tunnel: w213 -> [_]
          frame #0 {
            n100 = call "Manual.vi"("vi reference"=w224, "error in (no error)"=w225, "IOList_280"=w221) -> ("error out"=w223:errorcluster, "Out reference"=w222:refnum<vi>)  [unwired: 7 in]
          }
        }
      }
      frame "Report" {
      }
      frame "Testing" {
        n101 = Unbundle By Name(w232) -> ("DI List_280"=w231:string[])
        n102 = call "Program list Selection.vi"() -> ("Exit"=w233:bool, "String"=w235:string)  [unwired: 10 in]
        n103 = Concatenate Strings(w235, ".bin" ("string")) -> (w237:string)
        n104 = Build Path(base path=w234, name or relative path=w237) -> (appended path=w230:path)
        n105 = case shown="True" w233 {
          tunnel: w231 -> [_ w243]
          tunnel: w230 -> [_ w242]
          frame False {
          }
          frame True {
            n106 = call "Testing Mode.vi"("Filepath"=w242, "FeedBack Channel"=w243) -> ()  [unwired: 10 in]
          }
        }
      }
    }
    n107 = global write "Galobal variable_TI.vi" "Exit"(w59) -> ()
    n108 = invoke class="VI" method="FP.Open"(reference=w67, error in=w66, "Activate"=FALSE ("Activate?"), "State"=T19."Maximized") -> (reference out=w65:refnum<vi>, error out=w64:errorcluster)  [unwired: 1 in, 3 out]
  }
  n109 = disable-structure shown="Enabled" {
    frame Disabled {
    }
    frame Enabled {
    }
  }
